vi "Stop.vi"(8 "error in (no error)":errorcluster, 10 "Message in":refnum<class "StopMessage.lvclass">, 11 "BMC in":refnum<class "BMC.lvclass">) -> (0 "error out":errorcluster, 3 "BMC out":refnum<class "BMC.lvclass">)   [LabVIEW 2012, in "BMC.lvclass"]
doc: "This member function is called when the statemachine in the run.vi receives an 'stop' command. It relays the message to all observers of the component.\n\nOverride this member function in your derived class if you need additional stop functionality (but don't forget to call the parent method)."
uses:
  BMC.lvclass
  <vilib>/Distrio/Murmex/StopMessage/StopMessage.lvclass
  <vilib>/Distrio/Murmex/Murmex/Murmex.lvclass
panel:
  # "This method is called when the STOP\ntrigger is sent. \n\nOverride this method when your component needs to\nrespond to this trigger. \n\nCall parent for proper implementation"
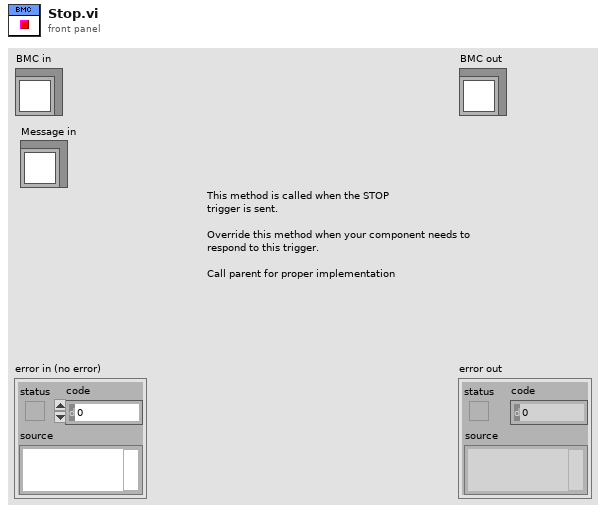
[diagram p1: front panel]
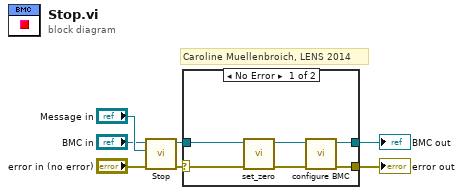
[diagram p0: block diagram]
diagram:
  # "Caroline Muellenbroich, LENS 2014"
  n1 = call-parent "Stop.vi"("error in (no error)"="error in (no error)", "Message in"="Message in", "Murmex in"="BMC in") -> ("error out"=w4:errorcluster, "Murmex out"=w3:refnum<class "BMC.lvclass">)  [unwired: 7 in]
  n2 = case shown="No Error" w4 {
    selector: w4 -> [w9 w14]
    tunnel: w3 -> [w8 w15]
    tunnel: [w13 w14] -> w2
    tunnel: [w12 w15] -> w1
    frame No Error {
      n3 = call-dynamic "set_zero.vi"("error in (no error)"=w9, "BMC in"=w8) -> ("error out"=w11:errorcluster, "BMC out"=w10:refnum<class "BMC.lvclass">)  [unwired: 8 in]
      n4 = call-dynamic "configure BMC.vi"("error in (no error)"=w11, "BMC in"=w10) -> ("error out"=w13:errorcluster, "BMC out"=w12:refnum<class "BMC.lvclass">)  [unwired: 8 in]
    }
    frame Error {
    }
  }
  "error out" <- w2
  "BMC out" <- w1
